vi "LogFile begrenzen.vi"(7 "max. Größe  in Byte":i64=31457280, 9 "Index (Eingang)":i16, 10 "Pfad (Eingang)":path, 11 "Pfad original (Eingang)":path) -> (1 "Index (Ausgang)":i16, 2 "Pfad (Ausgang)":path, 3 "Pfad original (Ausgang)":path)   [LabVIEW 2020, in "LogKonfig.lvlib"]
uses:
  LogKonfig.lvlib
panel:
  out "LogFile Daten out":string[][](array[string])
  in  "LogFile Daten in":string[][](array[string])
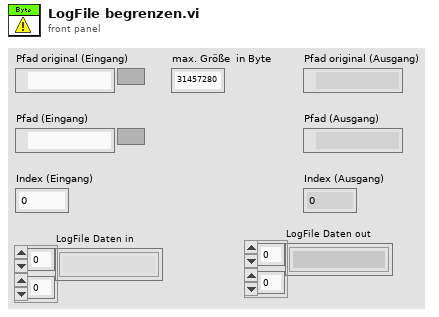
[diagram p1: front panel]
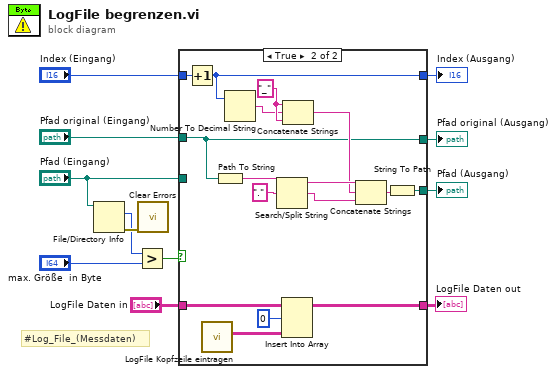
[diagram p0: block diagram]
diagram:
  # "#Log_File_(Messdaten)"
  n1 = File/Directory Info(path="Pfad (Eingang)") -> (size=w8:i64, error out=w9:errorcluster)  [unwired: 1 in, 5 out]
  n2 = Greater?(x=w8, y="max. Größe  in Byte") -> (0:w12:bool)
  n3 = call <vilib>:"Clear Errors.vi"("error in (no error)"=w9) -> ()  [unwired: 5 in, 2 out]
  n4 = case shown="True" w12 {
    tunnel: [w15 w27] -> w5
    tunnel: "Index (Eingang)" -> [w16 w23]
    tunnel: [w16 w22] -> w7
    tunnel: "Pfad (Eingang)" -> [w15 _]
    tunnel: "Pfad original (Eingang)" -> [w14 w21]
    tunnel: [w14 w21] -> w3
    tunnel: "LogFile Daten in" -> [w13 w20]
    tunnel: [w13 w19] -> w1
    frame False {
    }
    frame True {
      w26 = "_" ("String")
      n5 = Increment(x=w23) -> (x+1=w22:i16)
      n6 = call "LogFile Kopfzeile eintragen.vi"() -> ("LogFile Kopfzeile"=w18:string[][])  [unwired: 11 in]
      n7 = Path To String(path=w21) -> (string=w32:string)
      n8 = Number To Decimal String(number=w22) -> (decimal integer string=w25:string)  [unwired: 1 in]
      n9 = Search/Split String(string=w32, search string/char (-)="." ("Nach String/Zeichen suchen (-)")) -> (substring before match=w30:string, match + rest of string=w29:string)  [unwired: 1 in, 1 out]
      n10 = Insert Into Array(array=w20, index (row)=0 ("Index (Zeile)"), new element=w18) -> (w19:string[][])  [unwired: 1 in]
      n11 = Concatenate Strings(w26, w25, w26) -> (w24:string)
      n12 = Concatenate Strings(w30, w24, w29) -> (w28:string)
      n13 = String To Path(string=w28) -> (path=w27:path)
    }
  }
  "Pfad (Ausgang)" <- w5
  "Index (Ausgang)" <- w7
  "Pfad original (Ausgang)" <- w3
  "LogFile Daten out" <- w1
